vi "shooter bias fg.vi"(1 "Button 10 (dec)":bool, 2 "Button 11 (inc)":bool, 3 "Menu":T1) -> (0 "output":dbl)   [LabVIEW 2011]
uses:
  fg_typedef.ctl
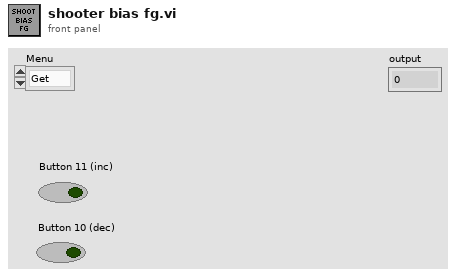
[diagram p1: front panel]
types:
  T1 = typedef "fg_typedef.ctl" = enum16{"Get", "Set"}
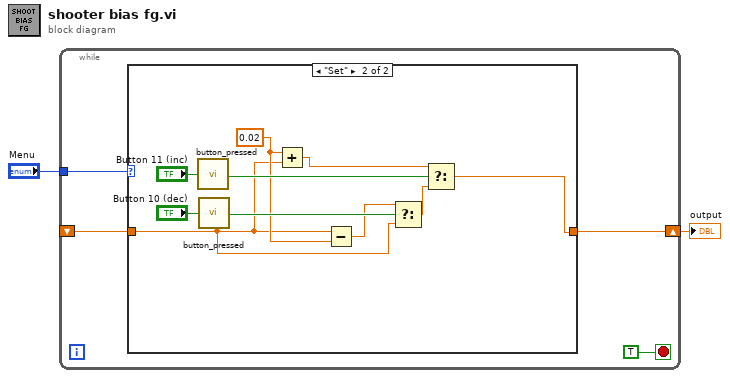
[diagram p0: block diagram]
diagram:
  n1 = while {
    shift-right: [w4] -> w1
    shift-left: _ -> [w3]
    tunnel: "Menu" -> [w5]
    stop <- TRUE stop-if-true
    n2 = case shown="\"Set\"" w5 {
      tunnel: [w7 w8] -> w4
      tunnel: w3 -> [w7 w9]
      frame "Get", Default {
      }
      frame "Set" {
        w11 = 0.02 ("y")
        n3 = call "button_pressed.vi"("Button In"="Button 11 (inc)") -> ("Button Pressed?"=w15:bool)
        n4 = call "button_pressed.vi"("Button In"="Button 10 (dec)") -> ("Button Pressed?"=w14:bool)
        n5 = Add(x=w11, y=w9) -> (x+y=w13:dbl)
        n6 = Subtract(x=w9, y=w11) -> (x-y=w12:dbl)
        n7 = Select(t=w12, s=w14, f=w9) -> (s? t:f=w10:dbl)
        n8 = Select(t=w13, s=w15, f=w10) -> (s? t:f=w8:dbl)
      }
    }
  }
  "output" <- w1
